vi "Load Sensor Locations.vi"(4 "Sensor Locations File":path=path "C:/Users/lane/Desktop/MuCool Test Area/Sensor.cfg") -> (1 "Sensor Locations":dbl[][](array[numeric]))   [LabVIEW 2013]
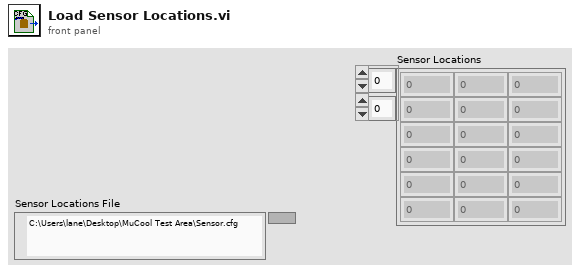
[diagram p1: front panel]
types:
  T1 = enum16{"big-endian, network order", "native, host order", "little-endian"}
  T2 = enum16{"open", "replace", "create", "open or create", "replace or create", "replace or create with confirmation"}
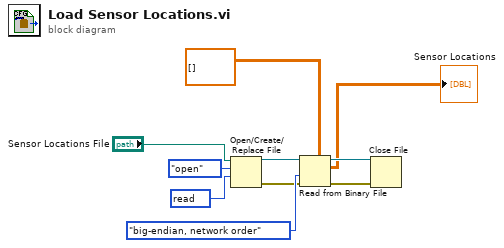
[diagram p0: block diagram]
diagram:
  w10 = u32 2147483648 items=["read"=2147483648, "write"=1073741824, "read & write"=3221225472, "execute"=536870912, "all"=268435456] ("desired access (read & write)")
  n1 = Open/Create/Replace File(file path (use dialog)="Sensor Locations File", operation (0:open)=T2."open", access (0:read/write)=w10) -> (refnum out=w6:refnum<file>, error out=w5:errorcluster)  [unwired: 3 in, 1 out]
  n2 = Read from Binary File(5:dbl[][] [] ("Array 2"), 8:w5, 9:T1."big-endian, network order" ("byte order (0:big-endian, network order)"), 11:w6) -> (0:w3:errorcluster, 2:→"Sensor Locations":dbl[][], 3:w4:refnum<file>)  [unwired: 2 in, 1 out]
  n3 = Close File(refnum=w4, error in=w3) -> ()  [unwired: 2 out]
